vi "Configure Serial Bus (IIC - Trigger).vi"(0 "VISA resource name":refnum<visa-resource-name>, 1 "Data Pattern (-1)":i32=-1, 2 "Data Qualifier (0: Equal)":i32(ring) items=["Equal", "Not Equal", "Less Than", "Greater Than"], 5 "Serial Bus Name (1: Serial Bus 1)":i32(ring)=1 items=["Serial Bus 1"=1, "Serial Bus 2"=2], 7 "Trigger Type (0: Start)":i32(ring) items=["Start", "Stop", "Read Data 7-bit", "Read Data2 7-bit", "Read EEPROM", "Write Data 7-bit", "Write Data2 7-bit", "Write Data 10-bit", "No ACK", "Address No ACK", "Restart", "Address", "Data No ACK"], 9 "Address (-1)":i32=-1, 11 "error in (no error)":errorcluster, 12 "Data 2 Pattern (-1)":dbl=-1.0) -> (4 "VISA resource name out":refnum<visa-resource-name>, 15 "error out":errorcluster)   [LabVIEW 2015, in "Agilent 2000 3000 X-Series.lvlib"]
doc: "Configures the trigger settings of IIC bus."
uses:
  <instrlib>/Agilent 2000 3000 X-Series/Agilent 2000 3000 X-Series.lvlib
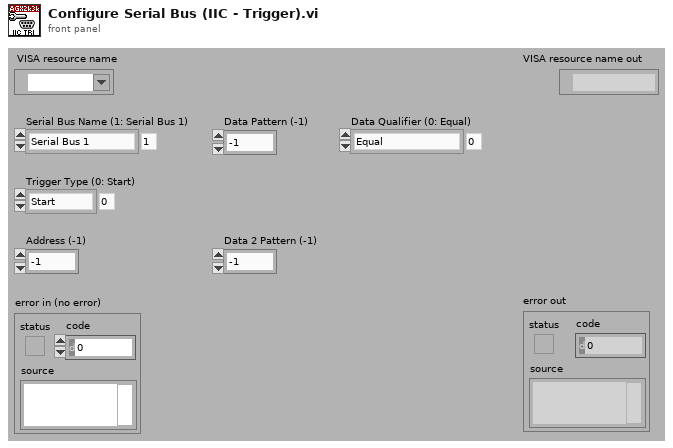
[diagram p1: front panel]
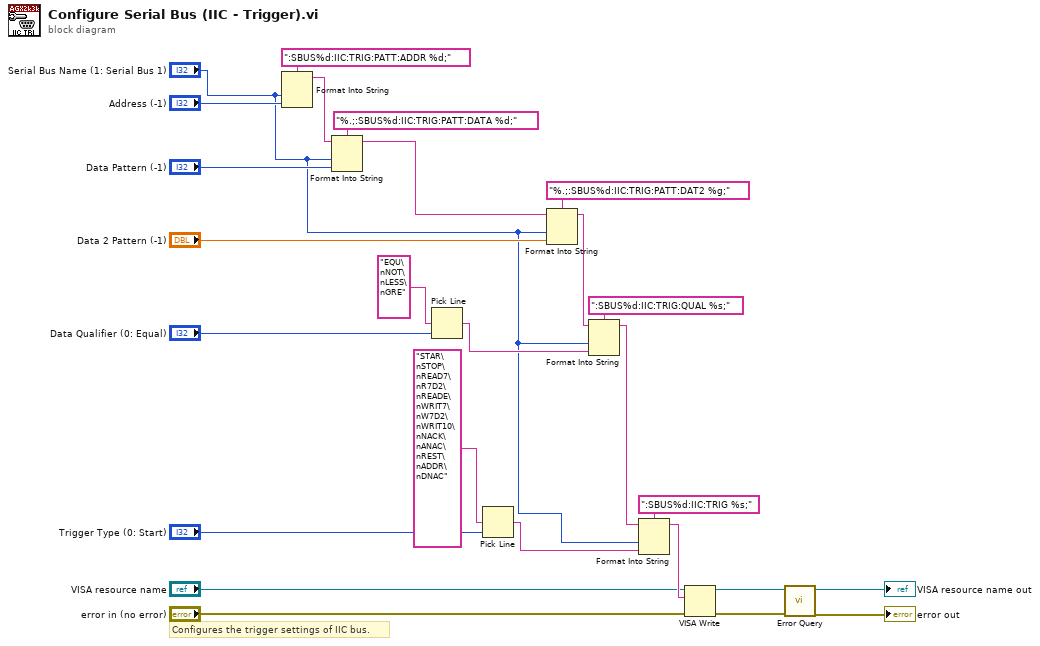
[diagram p0: block diagram]
diagram:
  # "Configures the trigger settings of IIC bus."
  n1 = Format Into String(format string=":SBUS%d:IIC:TRIG:PATT:ADDR %d;", "Serial Bus Name (1: Serial Bus 1)", "Address (-1)") -> (resulting string=w2:string)  [unwired: 2 in, 1 out]
  n2 = Format Into String(format string="%.;:SBUS%d:IIC:TRIG:PATT:DATA %d;", initial string=w2, "Serial Bus Name (1: Serial Bus 1)", "Data Pattern (-1)") -> (resulting string=w1:string)  [unwired: 1 in, 1 out]
  n3 = Pick Line(multi-line string="EQU\nNOT\nLESS\nGRE", line index="Data Qualifier (0: Equal)") -> (output string=w17:string)  [unwired: 1 out]
  n4 = Pick Line(multi-line string="STAR\nSTOP\nREAD7\nR7D2\nREADE\nWRIT7\nW7D2\nWRIT10\nNACK\nANAC\nREST\nADDR\nDNAC", line index="Trigger Type (0: Start)") -> (output string=w12:string)  [unwired: 1 out]
  n5 = Format Into String(format string="%.;:SBUS%d:IIC:TRIG:PATT:DAT2 %g;", initial string=w1, "Serial Bus Name (1: Serial Bus 1)", "Data 2 Pattern (-1)") -> (resulting string=w19:string)  [unwired: 1 in, 1 out]
  n6 = Format Into String(format string=":SBUS%d:IIC:TRIG:QUAL %s;", initial string=w19, "Serial Bus Name (1: Serial Bus 1)", w17) -> (resulting string=w14:string)  [unwired: 1 in, 1 out]
  n7 = Format Into String(format string=":SBUS%d:IIC:TRIG %s;", initial string=w14, "Serial Bus Name (1: Serial Bus 1)", w12) -> (resulting string=w11:string)  [unwired: 1 in, 1 out]
  n8 = VISA Write(VISA resource name="VISA resource name", write buffer=w11, error in (no error)="error in (no error)") -> (VISA resource name out=w8:refnum<visa-resource-name>, error out=w7:errorcluster)  [unwired: 1 out]
  n9 = call <instrlib>:"Error Query.vi"("error in (no error)"=w7, "VISA resource name"=w8) -> ("error out"=→"error out":errorcluster, "VISA resource name out"=→"VISA resource name out":refnum<visa-resource-name>)  [unwired: 8 out]
